vi "CPP-6068Special.vi"() -> (5 "Plug in titles":string[](array[string]), 7 "Plug in values":string[](array[string]))   [LabVIEW 2011]
uses:
  Globals/Meas_global.vi
  CPP/ProjectSpecific/6068-VeerTowers/MesowestParse/MetDataGlobal.vi
  Globals/Constants_global.vi
panel:
  in  "Marry-in Met Data?":bool
  out "Results":string[][](table)
  in  "OutputFile":path
  out "BlockStartTime":dbl format="%#_12f"
  in  "SearchBands":cluster{"Min":dbl, "Max":dbl, "Name":string}[](array[cluster])=[{"Min"=40.0, "Max"=70.0, "Name"="60Hz:Band"}, {"Min"=100.0, "Max"=140.0, "Name"="120Hz:Band"}, {"Min"=450.0, "Max"=510.0, "Name"="480Hz:Band"}, {"Min"=600.0, "Max"=680.0, "Name"="640Hz:Band"}, {"Min"=520.0, "Max"=590.0, "Name"="550Hz:Band"}]
  out "TimeRunStarted":dbl format="%^<%H:%M:%S\n%x %Z>T"
  out "Processing last block?":bool
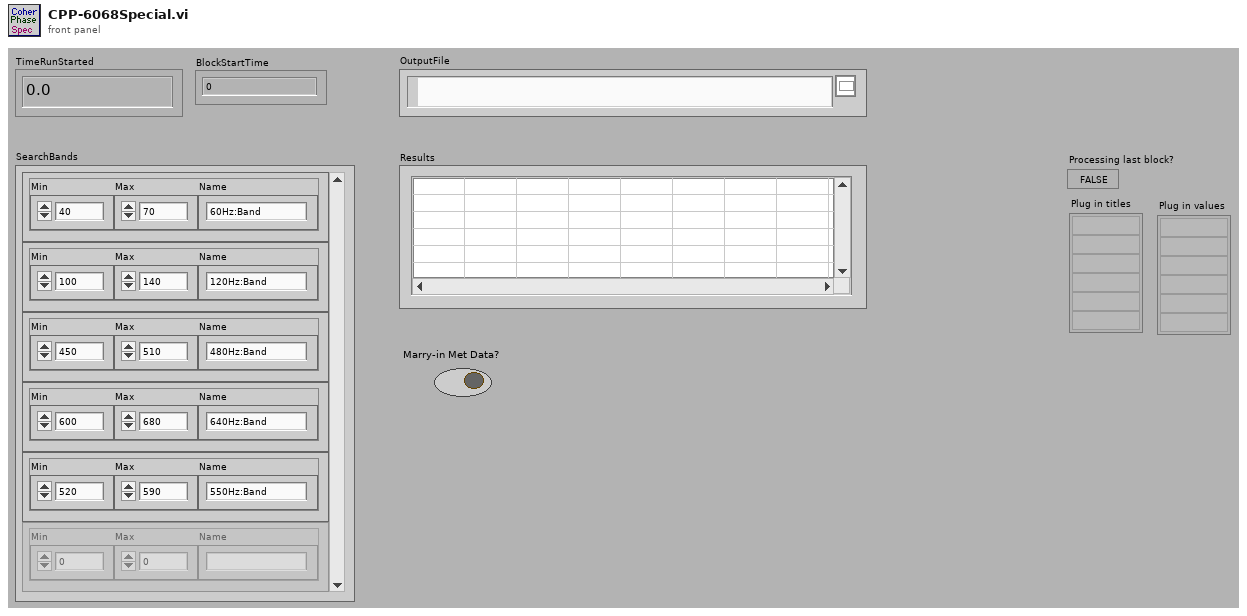
[diagram p1: front panel]
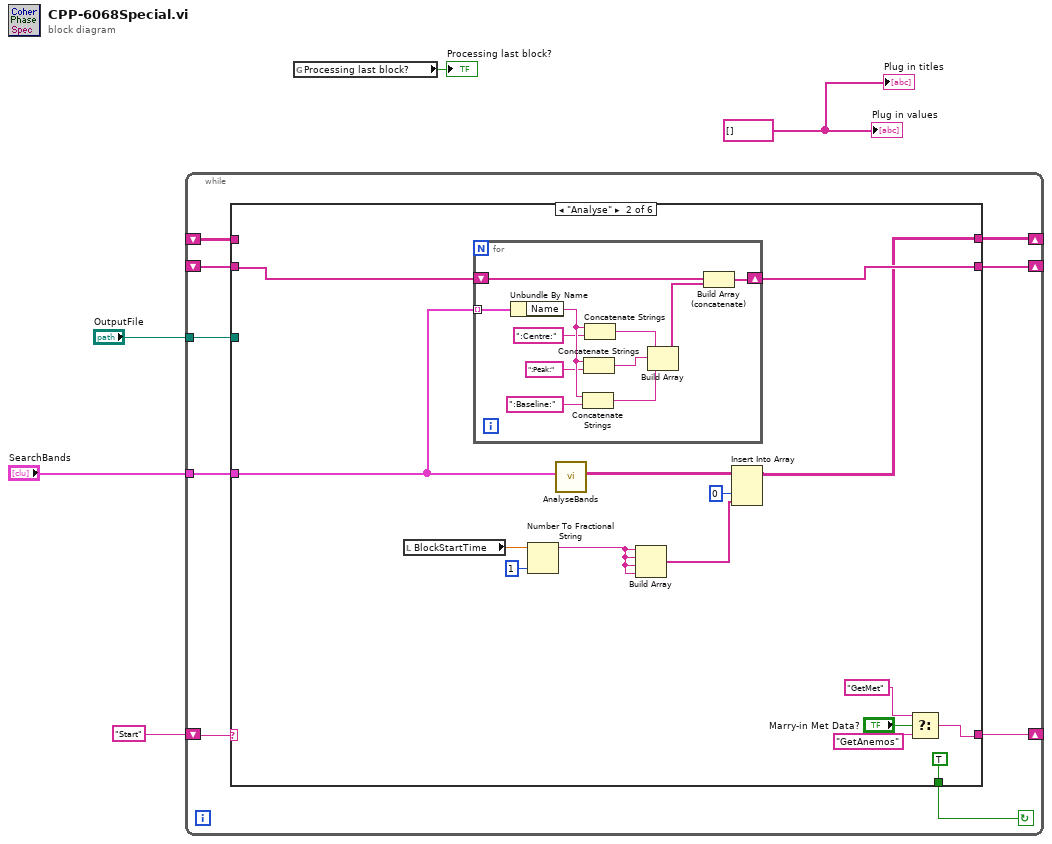
[diagram p0: block diagram]
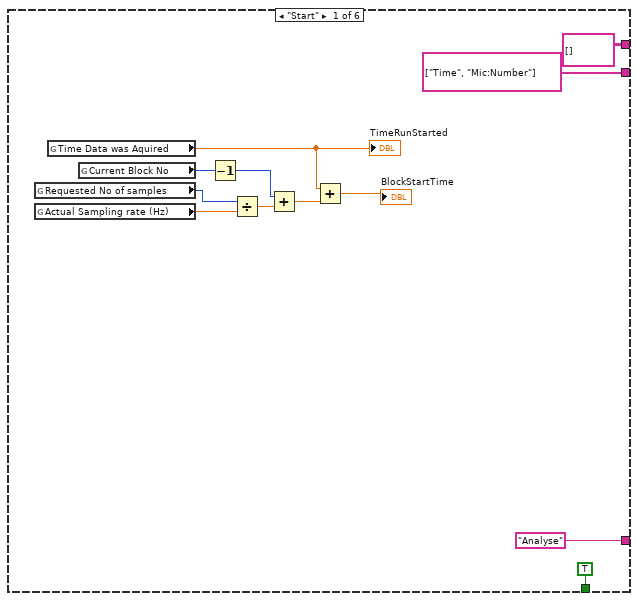
[diagram p2: hidden frame]
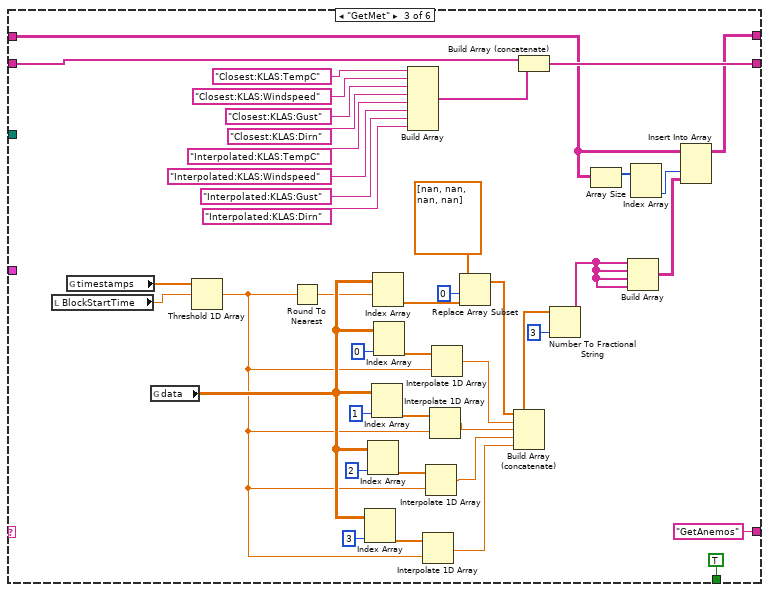
[diagram p3: hidden frame]
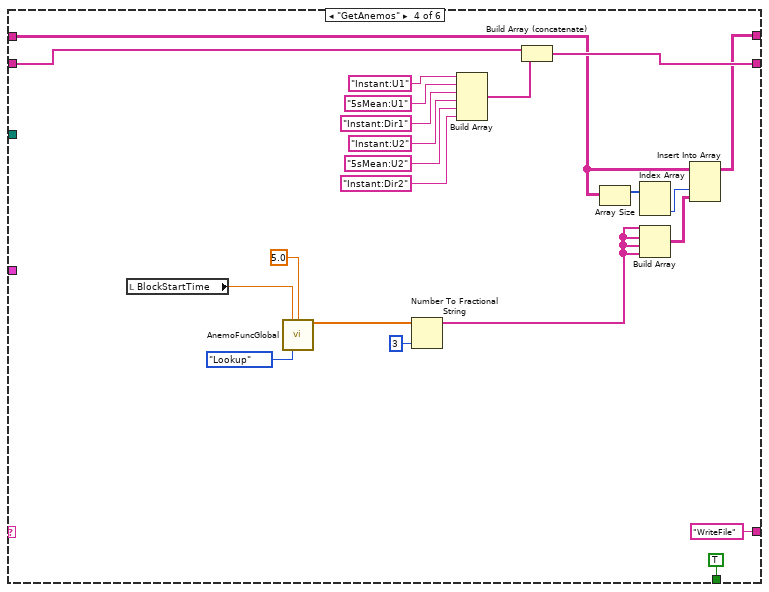
[diagram p4: hidden frame]
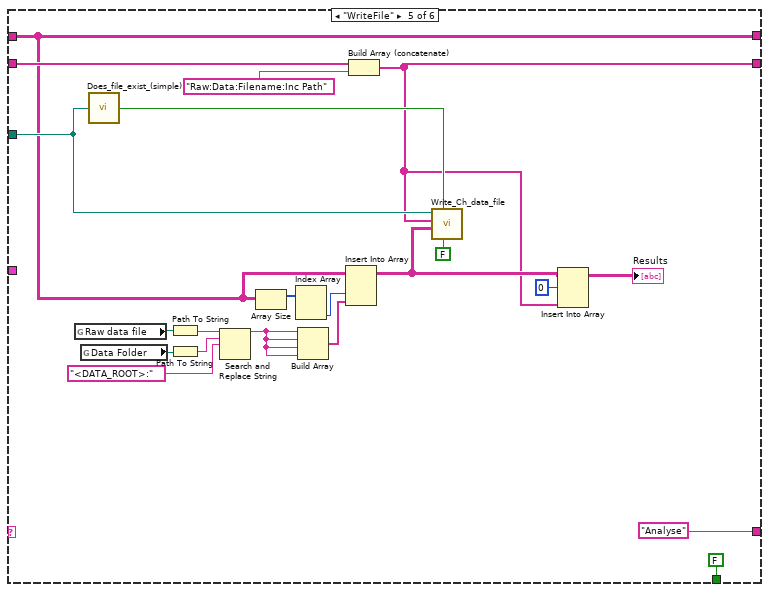
[diagram p5: hidden frame]
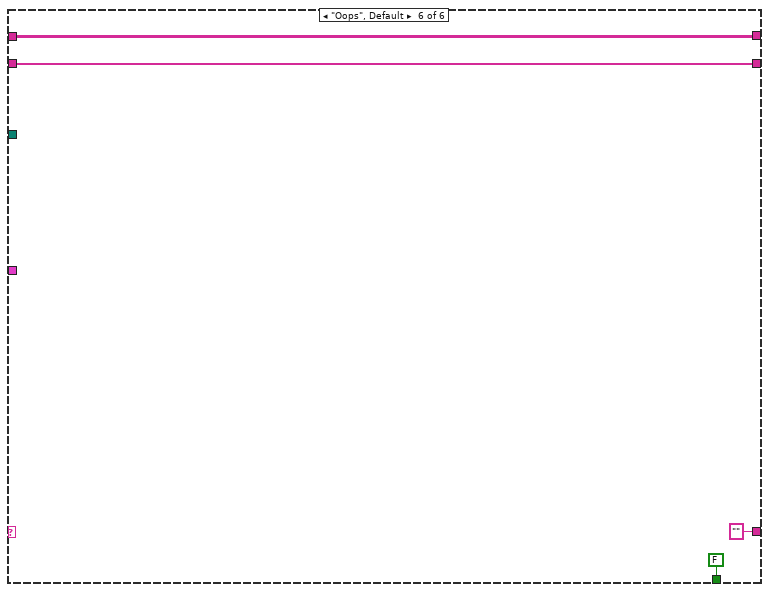
[diagram p6: hidden frame]
diagram:
  w4 = string[] [] ("Add in values")
  n1 = while {
    tunnel: "SearchBands" -> [w14]
    shift-right: [w12] -> _
    shift-left: "Start" -> [w13]
    shift-right: [w9] -> _
    shift-left: _ -> [w10]
    shift-right: [w7] -> _
    shift-left: _ -> [w8]
    tunnel: "OutputFile" -> [w6]
    stop <- w11 continue-if-true
    n2 = case shown="\"Analyse\"" w13 {
      tunnel: w14 -> [_ w36 _ _ _ _]
      tunnel: ["Analyse" w30 "GetAnemos" "WriteFile" "Analyse" ""] -> w12
      tunnel: [TRUE TRUE TRUE TRUE FALSE FALSE] -> w11
      tunnel: w10 -> [_ w35 w66 w107 w122 w139]
      tunnel: [string[] ["Time", "Mic:Number"] w34 w65 w106 w120 w139] -> w9
      tunnel: [string[][] [] ("Results") w33 w60 w103 w117 w138] -> w7
      tunnel: w8 -> [_ _ w62 w102 w117 w138]
      tunnel: w6 -> [_ _ _ _ w124 _]
      frame "Start" {
        n3 = global read "Meas_global.vi" "Requested No of samples"() -> (w24:i32)
        n4 = global read "Meas_global.vi" "Actual Sampling rate (Hz)"() -> (w23:dbl)
        n5 = global read "Meas_global.vi" "Time Data was Aquired"() -> (w19:dbl)
        "TimeRunStarted" <- w19
        n6 = global read "Meas_global.vi" "Current Block No"() -> (w25:i32)
        n7 = Decrement(x=w25) -> (x-1=w21:i32)
        n8 = Divide(x=w24, y=w23) -> (x/y=w22:dbl)
        n9 = Add(x=w21, y=w22) -> (x+y=w20:dbl)
        n10 = Add(x=w19, y=w20) -> (x+y=→"BlockStartTime":dbl)
      }
      frame "Analyse" {
        n11 = local read "BlockStartTime"() -> (w37:dbl)
        n12 = for {
          shift-right: [w44] -> w34
          shift-left: w35 -> [w42]
          tunnel: w36 -> [w52] mode=indexing
          n13 = Unbundle By Name(w52) -> ("Name"=w51:string)
          n14 = Concatenate Strings(w51, ":Baseline:" ("string")) -> (w45:string)
          n15 = Concatenate Strings(w51, ":Peak:" ("string")) -> (w46:string)
          n16 = Concatenate Strings(w51, ":Centre:" ("string")) -> (w47:string)
          n17 = Build Array(w47, w46, w45) -> (w43:string[])
          n18 = Build Array (concatenate)(w42, w43) -> (w44:string[])
        }
        n19 = Number To Fractional String(number=w37, precision (6)=i16 1) -> (F-format string=w32:string)  [unwired: 2 in]
        n20 = call "AnalyseBands.vi"("SearchBands"=w36) -> ("Results"=w41:string[][])  [unwired: 10 in]
        n21 = Build Array(w32, w32, w32, w32) -> (w40:string[])
        n22 = Insert Into Array(array=w41, index (col)=0 ("disabled index (col)"), new element=w40) -> (w33:string[][])  [unwired: 1 in]
        n23 = Select(t="GetMet", s="Marry-in Met Data?", f="GetAnemos") -> (s? t:f=w30:string)
      }
      frame "GetMet" {
        n24 = local read "BlockStartTime"() -> (w91:dbl)
        n25 = global read "MetDataGlobal.vi" "timestamps"() -> (w94:dbl[])
        n26 = global read "MetDataGlobal.vi" "data"() -> (w78:dbl[][])
        n27 = Threshold 1D Array(2:w91, 3:w94) -> (0:w77:dbl)  [unwired: 1 in]
        n28 = Round To Nearest(number=w77) -> (nearest integer value=w76:dbl)
        n29 = Index Array(array=w78, index (col)=3 ("disabled index (col)")) -> (element=w84:dbl[])  [unwired: 1 in]
        n30 = Index Array(array=w78, index (col)=2 ("disabled index (col)")) -> (element=w85:dbl[])  [unwired: 1 in]
        n31 = Index Array(array=w78, index (col)=1 ("disabled index (col)")) -> (element=w88:dbl[])  [unwired: 1 in]
        n32 = Index Array(array=w78, index (row)=w76) -> (element=w57:dbl[])  [unwired: 1 in]
        n33 = Index Array(array=w78, index (col)=0 ("disabled index (col)")) -> (element=w89:dbl[])  [unwired: 1 in]
        n34 = Build Array("Closest:KLAS:TempC", "Closest:KLAS:Windspeed", "Closest:KLAS:Gust", "Closest:KLAS:Dirn", "Interpolated:KLAS:TempC", "Interpolated:KLAS:Windspeed", "Interpolated:KLAS:Gust", "Interpolated:KLAS:Dirn") -> (w67:string[])
        n35 = Interpolate 1D Array(1:w77, 2:w84) -> (0:w79:dbl)
        n36 = Interpolate 1D Array(1:w77, 2:w85) -> (0:w80:dbl)
        n37 = Interpolate 1D Array(1:w77, 2:w88) -> (0:w81:dbl)
        n38 = Interpolate 1D Array(1:w77, 2:w89) -> (0:w82:dbl)
        n39 = Replace Array Subset(array=dbl[] [nan, nan, nan, nan], new element=w57, index=0) -> (w58:dbl[])
        n40 = Build Array (concatenate)(w58, w82, w81, w80, w79) -> (w64:dbl[])
        n41 = Build Array (concatenate)(w66, w67) -> (w65:string[])
        n42 = Number To Fractional String(number=w64, precision (6)=i16 3) -> (F-format string=w54:string[])  [unwired: 2 in]
        n43 = Array Size(array=w62) -> (size(s)=w61:i32[])
        n44 = Build Array(w54, w54, w54, w54) -> (w63:string[][])
        n45 = Index Array(array=w61) -> (element #2=w59:i32)  [unwired: 2 in, 1 out]
        n46 = Insert Into Array(array=w62, index (col)=w59, new element=w63) -> (w60:string[][])  [unwired: 1 in]
      }
      frame "GetAnemos" {
        n47 = local read "BlockStartTime"() -> (w101:dbl)
        n48 = call "AnemoFuncGlobal.vi"("searchValue"=w101, "history(samples)"=5.0 ("fractional index or x"), "Mode"=enum16{"Overwrite", "Append", "Read", "Lookup"}."Lookup") -> ("results"=w99:dbl[])  [unwired: 12 in]
        n49 = Number To Fractional String(number=w99, precision (6)=i16 3) -> (F-format string=w96:string[])  [unwired: 2 in]
        n50 = Build Array("Instant:U1", "5sMean:U1", "Instant:Dir1", "Instant:U2", "5sMean:U2", "Instant:Dir2") -> (w108:string[])
        n51 = Build Array (concatenate)(w107, w108) -> (w106:string[])
        n52 = Array Size(array=w102) -> (size(s)=w105:i32[])
        n53 = Index Array(array=w105) -> (element #2=w104:i32)  [unwired: 2 in, 1 out]
        n54 = Build Array(w96, w96, w96, w96) -> (w97:string[][])
        n55 = Insert Into Array(array=w102, index (col)=w104, new element=w97) -> (w103:string[][])  [unwired: 1 in]
      }
      frame "WriteFile" {
        n56 = global read "Meas_global.vi" "Raw data file"() -> (w130:path)
        n57 = global read "Constants_global.vi" "Data Folder"() -> (w129:path)
        n58 = call "Does_file_exist_(simple).vi"("Pathname"=w124) -> ("exists?"=w135:bool)
        n59 = Path To String(path=w130) -> (string=w128:string)
        n60 = Path To String(path=w129) -> (string=w127:string)
        n61 = Search and Replace String(input string=w128, search string=w127, replace string="<DATA_ROOT>:" ("replace string (\"\")")) -> (result string=w126:string)  [unwired: 5 in, 3 out]
        n62 = Array Size(array=w117) -> (size(s)=w132:i32[])
        n63 = Index Array(array=w132) -> (element #2=w131:i32)  [unwired: 2 in, 1 out]
        n64 = Build Array(w126, w126, w126, w126) -> (w133:string[])
        n65 = Insert Into Array(array=w117, index (col)=w131, new element=w133) -> (w121:string[][])  [unwired: 1 in]
        n66 = Build Array (concatenate)(w122, "Raw:Data:Filename:Inc Path") -> (w120:string[])
        n67 = call "Write_Ch_data_file.vi"("Lock File"=FALSE, "exists?"=w135, "Channel Values"=w121, "Channel names"=w120, "Filename"=w124) -> ()  [unwired: 7 in]
        n68 = Insert Into Array(array=w121, index (row)=0, new element=w120) -> (→"Results":string[][])  [unwired: 1 in]
      }
      frame "Oops", Default {
      }
    }
  }
  n69 = global read "Meas_global.vi" "Processing last block?"() -> (→"Processing last block?":bool)
  "Plug in titles" <- w4
  "Plug in values" <- w4
